vi "Delete.vi"(8 "error in (no error)":errorcluster, 11 "Value in":refnum<class "Value.lvclass">) -> (0 "error out":errorcluster)   [LabVIEW 2020, in "Value.lvlib" / "Value.lvclass"]
uses:
  Value.lvclass
  Value.lvclass/Value.ctl
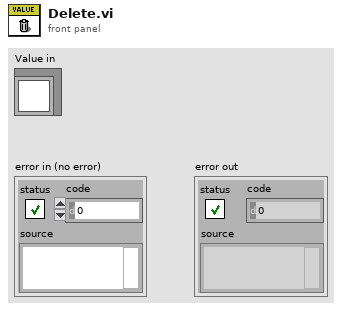
[diagram p1: front panel]
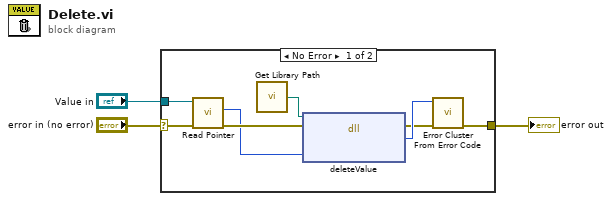
[diagram p0: block diagram]
diagram:
  n1 = case shown="No Error" "error in (no error)" {
    selector: "error in (no error)" -> [w11 w12]
    tunnel: "Value in" -> [w10 _]
    tunnel: [w7 w12] -> w1
    frame No Error {
      n2 = call-dynamic "Read Pointer.vi"("error in (no error)"=w11, "Value in"=w10) -> ("error out"=w9:errorcluster, "pointer"=w8:i64)  [unwired: 7 in, 1 out]
      n3 = call "Get Library Path.vi"() -> ("Path"=w4:path)  [unwired: 1 in]
      n4 = dll-call lib="?" fn="deleteValue"(path in=w4, error in=w9, "value"=w8) -> (error out=w5:errorcluster, "ret code"=w6:i32)  [unwired: 2 in, 1 out]
      n5 = call <vilib>:"Error Cluster From Error Code.vi"("error in (no error)"=w5, "error code (0)"=w6) -> ("error out"=w7:errorcluster)  [unwired: 7 in]
    }
    frame Error {
    }
  }
  "error out" <- w1
